vi "PID Init.vi"(10 "Output Range":cluster{"output high":dbl, "output low":dbl}={"output high"=1.0, "output low"=-1.0}, 11 "PIDF Gains":cluster{"Kp":dbl, "Ki":dbl, "Kd":dbl, "Kf":dbl}={"Kp"=5.0, "Ki"=0.0, "Kd"=0.0, "Kf"=0.0} {"Kf" format="%.3f"; "Kd" format="%.3f"; "Ki" format="%.3f"; "Kp" format="%.3f"}) -> (3 "PID Ref":refnum<data-value>)   [LabVIEW 2019]
uses:
  Typedef/PID Controller State.ctl
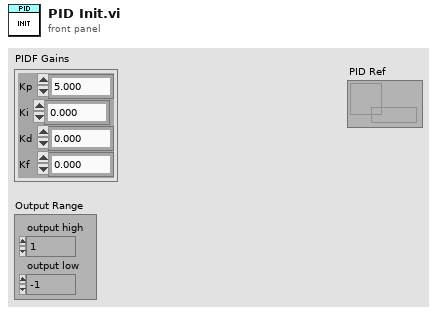
[diagram p1: front panel]
types:
  T1 = typedef "PID Controller State.ctl" = cluster{"PIDF Gains":cluster{"Kp":dbl, "Ki":dbl, "Kd":dbl, "Kf":dbl}, "Output Range":cluster{"output high":dbl, "output low":dbl}, "Profiled?":bool, "PID State":cluster{"iState":dbl, "dState":dbl, "Error [n-1]":dbl, "Output":dbl}, "Setpoint":dbl, "Profiled State":cluster{"Position":dbl, "Velocity":dbl}, "Profiled Contraints":cluster{"Max Velocity":dbl, "Max Acceleration":dbl}}
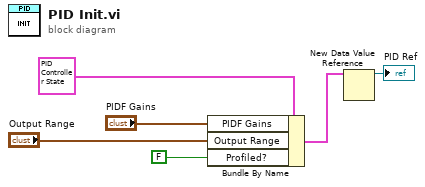
[diagram p0: block diagram]
diagram:
  n1 = Bundle By Name(cluster=T1 {"PIDF Gains"={"Kp"=0.0, "Ki"=0.0, "Kd"=0.0, "Kf"=0.0}, "Output Range"={"output high"=1.0, "output low"=-1.0}, "Profiled?"=FALSE, "PID State"={"iState"=0.0, "dState"=0.0, "Error [n-1]"=0.0, "Output"=0.0}, "Setpoint"=0.0, "Profiled State"={"Position"=0.0, "Velocity"=0.0}, "Profiled Contraints"={"Max Velocity"=0.0, "Max Acceleration"=0.0}}, "PIDF Gains"="PIDF Gains", "Output Range"="Output Range", "Profiled?"=FALSE) -> (w2:T1)
  n2 = New Data Value Reference(data value=w2) -> (data value reference=→"PID Ref":refnum<data-value>)  [unwired: 1 in, 1 out]
